vi "galvoWriteOpen.vi"   [LabVIEW 2017]
uses:
  globalDevices.vi
  <vilib>/DAQmx/create/channels.llb/DAQmx Create Channel (AO-Voltage-Basic).vi
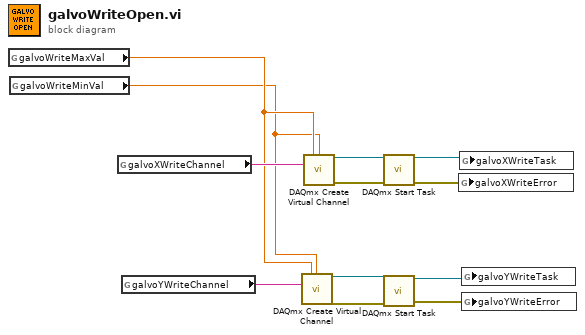
[diagram p0: block diagram]
diagram:
  n1 = global read "globalDevices.vi" "galvoWriteMaxVal"() -> (w2:dbl)
  n2 = global read "globalDevices.vi" "galvoWriteMinVal"() -> (w1:dbl)
  n3 = global read "globalDevices.vi" "galvoXWriteChannel"() -> (w12:tag)
  n4 = global read "globalDevices.vi" "galvoYWriteChannel"() -> (w11:tag)
  n5 = call-poly <vilib>:"DAQmx Create Virtual Channel.vi"("maximum value"=w2, "minimum value"=w1, "physical channels"=w11) -> ("task out"=w8:refnum<k21>, "error out"=w7:errorcluster)  [unwired: 11 in]
  n6 = call-poly <vilib>:"DAQmx Create Virtual Channel.vi"("maximum value"=w2, "minimum value"=w1, "physical channels"=w12) -> ("task out"=w10:refnum<k21>, "error out"=w9:errorcluster)  [unwired: 11 in]
  n7 = call <vilib>:"DAQmx Start Task.vi"("task/channels in"=w10, "error in"=w9) -> ("task out"=w6:refnum<k21>, "error out"=w5:errorcluster)  [unwired: 12 in]
  n8 = call <vilib>:"DAQmx Start Task.vi"("task/channels in"=w8, "error in"=w7) -> ("task out"=w4:refnum<k21>, "error out"=w3:errorcluster)  [unwired: 12 in]
  n9 = global write "globalDevices.vi" "galvoXWriteError"(w5) -> ()
  n10 = global write "globalDevices.vi" "galvoXWriteTask"(w6) -> ()
  n11 = global write "globalDevices.vi" "galvoYWriteTask"(w4) -> ()
  n12 = global write "globalDevices.vi" "galvoYWriteError"(w3) -> ()
